vi "RegexTester.vi"() -> ()   [LabVIEW 2017]
uses:
  <vilib>/regexp/Match Regular Expression.xnode
panel:
  out "before match":string
  out "Output":string
  in  "regular expression":string="Exec: .*\n"
  in  "String":string
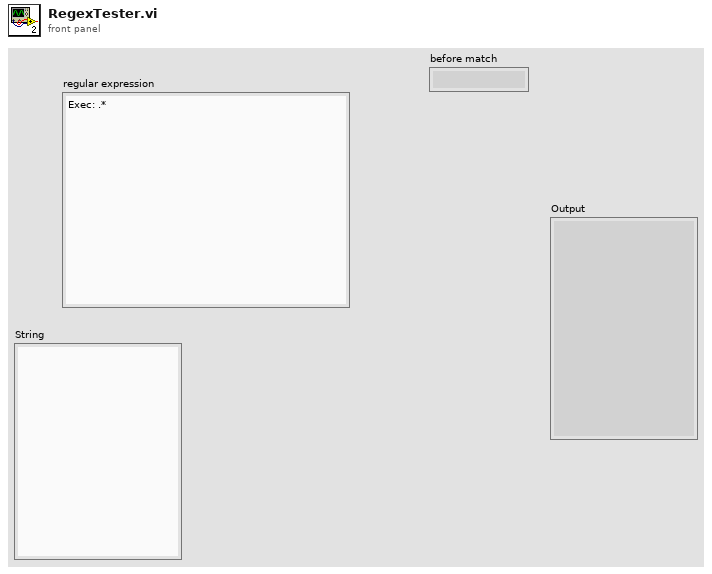
[diagram p1: front panel]
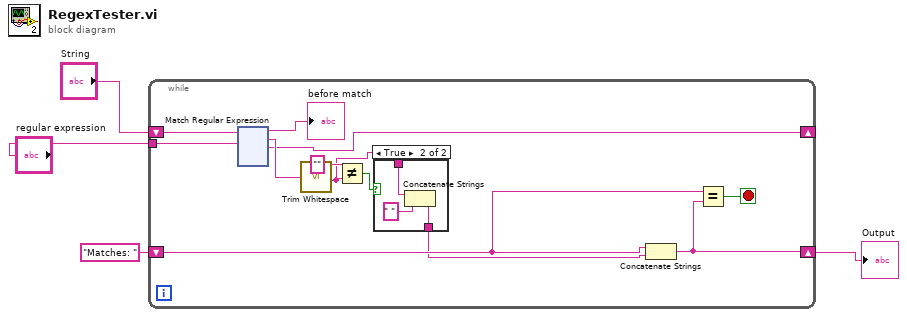
[diagram p0: block diagram]
diagram:
  n1 = while {
    shift-right: [w12] -> _
    shift-left: "String" -> [w16]
    tunnel: "regular expression" -> [w14]
    shift-right: [w11] -> w1
    shift-left: "Matches: " -> [w10]
    stop <- w15 stop-if-true
    n2 = xnode "Match Regular Expression"("input string"=w16, "regular expression"=w14) -> ("before match"=→"before match":string, "whole match"=w13:string, "after match"=w12:string)  [unwired: 4 in, 2 out]
    n3 = call <vilib>:"Trim Whitespace.vi"("string"=w13) -> ("trimmed string"=w7:string)  [unwired: 1 in]
    n4 = Not Equal?(x="", y=w7) -> (x != y?=w8:bool)
    n5 = case shown="True" w8 {
      tunnel: w7 -> [w17 w19]
      tunnel: [w17 w18] -> w6
      frame False {
      }
      frame True {
        n6 = Concatenate Strings(w19, " " ("string")) -> (w18:string)
      }
    }
    n7 = Concatenate Strings(w10, w6) -> (w11:string)
    n8 = Equal?(x=w10, y=w11) -> (x = y?=w15:bool)
  }
  "Output" <- w1
